vi "Verify Combinations.vi"(5 "Label":string, 7 "Approval Tests.lvlib:Options.lvclass":refnum<class "Options.lvclass">, 8 "error in":errorcluster, 9 "ctl label -> value var[]":map{string, variant[]}(c390), 10 "VI Refnum":refnum<vi>) -> (0 "error out":errorcluster, 1 "Failure Message":string, 2 "Passed?":bool)   [LabVIEW 2020, in "Approval Tests.lvlib"]
doc: "This is similar to the verify parameterized (in fact it calls it behind the scenes). Instead of specifying each set of parameters, you specify a single map which maps each control label to an array of variant values (there is a utility vi, \"array to array of variants.vim) to assist with this. From this, the verify function calculates each set of parameters from all the possible combinations and verifyies each combination."
uses:
  Approval Tests.lvlib
  Options/Options.lvclass
  Options/Options.lvclass/Options.ctl
  Naming Data/Naming Data.lvclass/Naming Data.ctl
  Naming Data/Read Test VI Name.vi
  Naming Data/Write Test VI Name.vi
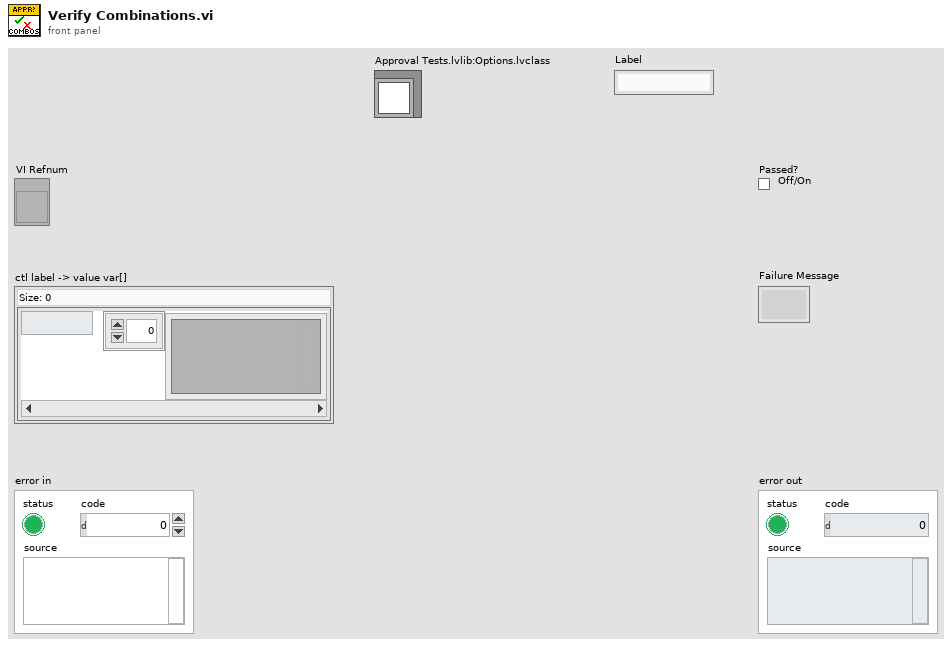
[diagram p1: front panel]
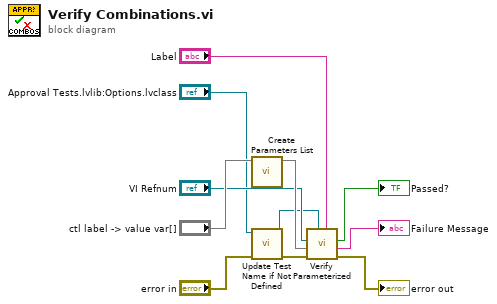
[diagram p0: block diagram]
diagram:
  n1 = call "Create Parameters List.vi"("ctl label -> value var[]"="ctl label -> value var[]") -> ("Set of ctl label -> value var combos"=w5:set{map{string, variant}})  [unwired: 10 in]
  n2 = call "Update Test Name if Not Defined.vi"("error in"="error in", "Options in"="Approval Tests.lvlib:Options.lvclass") -> ("error out"=w9:errorcluster, "Options out"=w2:refnum<class "Options.lvclass">)  [unwired: 8 in]
  n3 = call "Verify Parameterized.vi"("Label"="Label", "Approval Tests.lvlib:Options.lvclass"=w2, "error in"=w9, "Set of ctl label -> value var"=w5, "VI in"="VI Refnum") -> ("error out"=→"error out":errorcluster, "Failure Message"=→"Failure Message":string, "Passed?"=→"Passed?":bool)  [unwired: 4 in]
